vi "P4CMD File Status.vi"(8 "error in (no error)":errorcluster, 10 "files":path[](array[path]), 11 "source control reference in":T2) -> (0 "error out":errorcluster, 1 "file status":T1[](array[typedef]), 2 "status message":string, 3 "source control reference out":T2, 4 "files status flags":i32[](array[numeric]))   [LabVIEW 2020, in "NI_SCC_P4CMD.lvlib"]
uses:
  <vilib>/SourceControl/Providers/P4CMD/NI_SCC_P4CMD.lvlib
  <vilib>/SourceControl/sccapi/SCCAPI Refnum.ctl
  <vilib>/SourceControl/sccapi/SCCAPI SCC File Status.ctl
  <vilib>/SourceControl/support/SCCSup Message Strings GLBL.vi
  <vilib>/SourceControl/sccapi/NI_SCC.lvlib
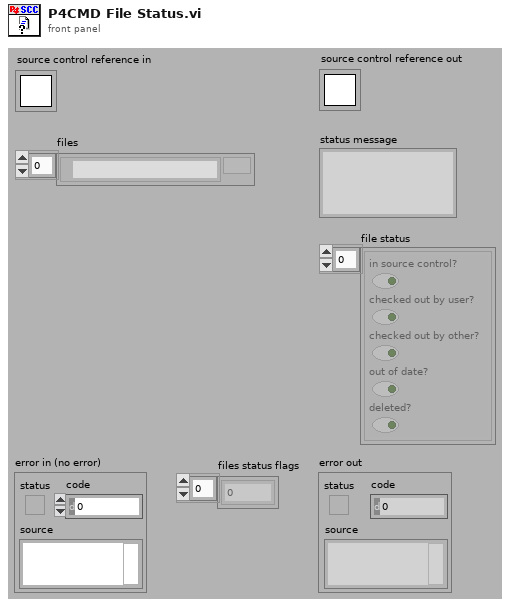
[diagram p1: front panel]
types:
  T1 = typedef "NI_SCC.lvlib/SCCAPI SCC File Status.ctl" = cluster{"in source control?":bool, "checked out by user?":bool, "checked out by other?":bool, "out of date?":bool, "deleted?":bool}
  T2 = typedef "NI_SCC.lvlib/SCCAPI Refnum.ctl" = refnum<k1>
  T3 = typedef "NI_SCC_P4CMD.lvlib/P4CMD SCC File Status.ctl" = cluster{"source controlled":bool, "open by user":bool, "open by other":bool, "out of date":bool, "deleted":bool, "locked by user":bool, "locked by other":bool, "open for add by user":bool, "open for delete by user":bool}
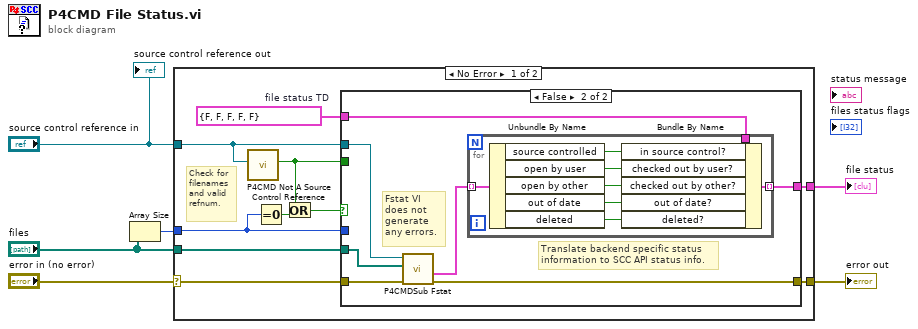
[diagram p0: block diagram]
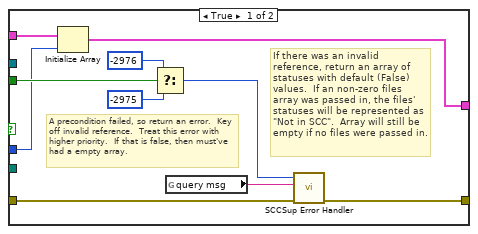
[diagram p2: hidden frame]
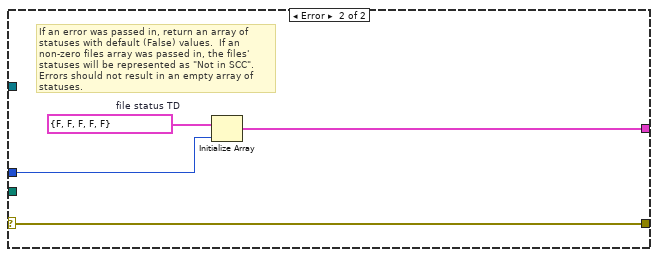
[diagram p3: hidden frame]
diagram:
  n1 = Array Size(array="files") -> (size(s)=w1:i32)
  n2 = case shown="No Error" "error in (no error)" {
    selector: "error in (no error)" -> [w10 w45]
    tunnel: [w9 w45] -> w5
    tunnel: "source control reference in" -> [w14 _]
    tunnel: "files" -> [w13 _]
    tunnel: [w16 w43] -> w3
    tunnel: w1 -> [w7 w44]
    frame No Error {
      w8 = T1 {"in source control?"=FALSE, "checked out by user?"=FALSE, "checked out by other?"=FALSE, "out of date?"=FALSE, "deleted?"=FALSE}  # file status TD
      # "Check for filenames and valid refnum."
      n3 = call <vilib>:"P4CMD Not A Source Control Reference.vi"("source control reference in"=w14) -> ("not a source control reference?"=w11:bool)  [unwired: 9 in, 1 out]
      n4 = Equal To 0?(x=w7) -> (x = 0?=w15:bool)
      n5 = Or(x=w11, y=w15) -> (x .or. y?=w12:bool)
      n6 = case shown="False" w12 {
        tunnel: w14 -> [_ w29]
        tunnel: w13 -> [_ w30]
        tunnel: [w18 w31] -> w16
        tunnel: w11 -> [w24 _]
        tunnel: w10 -> [w21 w33]
        tunnel: [w22 w28] -> w9
        tunnel: w7 -> [w19 _]
        tunnel: w8 -> [w20 w27]
        frame True {
          # "If there was an invalid reference, return an array of statuses with default (False) values.  If an non-zero files array was passed in, the files' statuses will be represented as \"Not in SCC\".  Array will still be empty if no files were passed in."
          # "A precondition failed, so return an error.  Key off invalid reference.  Treat this error with higher priority.  If that is false, then must've had a empty array."
          n7 = Initialize Array(w20, w19) -> (w18:T1[])
          n8 = Select(t=-2976 ("result"), s=w24, f=-2975 ("result")) -> (s? t:f=w23:i32)
          n9 = global read "SCCSup Message Strings GLBL.vi" "query msg"() -> (w17:string)
          n10 = call <vilib>:"SCCSup Error Handler.vi"("error in (no error)"=w21, "operation message"=w17, "scc error code"=w23) -> ("error out"=w22:errorcluster)  [unwired: 8 in]
        }
        frame False {
          # "Fstat VI  does not generate any errors."
          # "Translate backend specific status information to SCC API status info."
          n11 = call <vilib>:"P4CMDSub Fstat.vi"("error in (no error)"=w33, "files"=w30, "source control reference in"=w29) -> ("error out"=w28:errorcluster, "files status"=w32:T3[])  [unwired: 5 in, 2 out]
          n12 = for {
            tunnel: w27 -> [w41]
            tunnel: w32 -> [w39] mode=indexing
            tunnel: [w40] -> w31 mode=indexing
            n13 = Unbundle By Name(w39) -> ("source controlled"=w38:bool, "open by user"=w37:bool, "open by other"=w36:bool, "out of date"=w35:bool, "deleted"=w34:bool)
            n14 = Bundle By Name(cluster=w41, "in source control?"=w38, "checked out by user?"=w37, "checked out by other?"=w36, "out of date?"=w35, "deleted?"=w34) -> (w40:T1)
          }
        }
      }
    }
    frame Error {
      w42 = T1 {"in source control?"=FALSE, "checked out by user?"=FALSE, "checked out by other?"=FALSE, "out of date?"=FALSE, "deleted?"=FALSE}  # file status TD
      # "If an error was passed in, return an array of statuses with default (False) values.  If an non-zero files array was passed in, the files' statuses will be represented as \"Not in SCC\".  Errors should not result in an empty array of statuses."
      n15 = Initialize Array(w42, w44) -> (w43:T1[])
    }
  }
  "error out" <- w5
  "file status" <- w3
  "source control reference out" <- "source control reference in"
